vi "Pause.vi"(8 "error in (no error)":errorcluster, 11 "Ismatech 3 Channel Settings In":T1={"VISA resource name"="", "Pump Number"=1, "Channel Number"=0, "Simulated?"=TRUE, "Reverse?"=FALSE} {"Channel Number" min=0 max=3; "Pump Number" min=1 max=9}) -> (0 "error out":errorcluster, 1 "Connection Error":bool, 2 "5 Fails":bool, 3 "Ismatech 3 Channel Settings Out":T1={"VISA resource name"="", "Pump Number"=1, "Channel Number"=0, "Simulated?"=TRUE, "Reverse?"=FALSE} {"Channel Number" min=0 max=3; "Pump Number" min=1 max=9})   [LabVIEW 2018, in "Ismatec 4308.lvlib"]
uses:
  Ismatec 4308.lvlib
  Ismatec 4083.ctl
  support/Support Library.lvlib
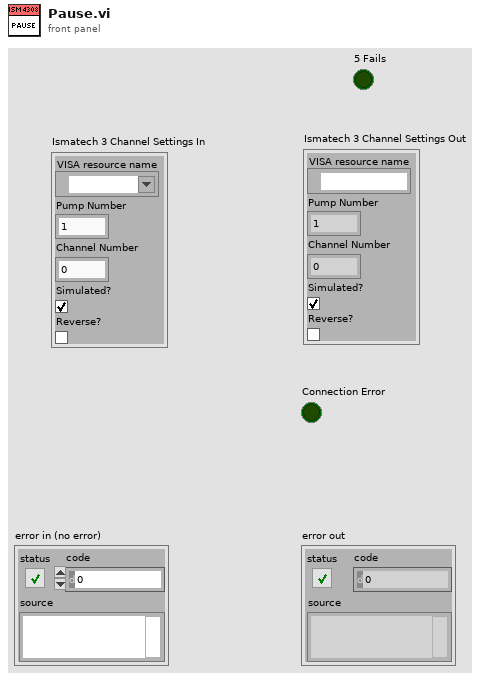
[diagram p1: front panel]
types:
  T1 = typedef "Ismatec 4308.lvlib/Ismatec 4083.ctl" = cluster{"VISA resource name":refnum<visa-resource-name>, "Pump Number":i16, "Channel Number":i16, "Simulated?":bool, "Reverse?":bool}
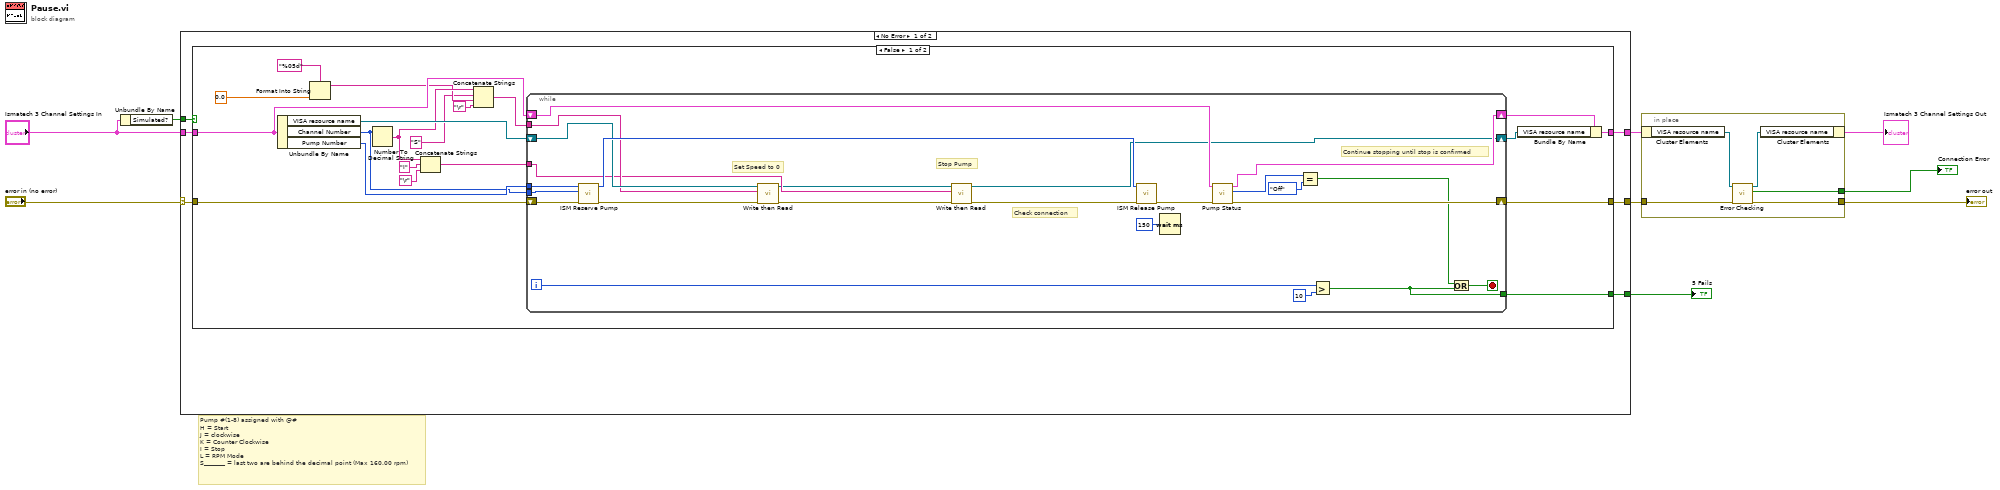
[diagram p0: block diagram]
diagram:
  # "Pump #(1-8) assigned with @#\nH = Start\nJ = clockwise\nK = Counter Clockwise\nI = Stop\nL = RPM Mode\nS_______ = last two are behind the decimal point (Max 160.00 rpm)"
  n1 = Unbundle By Name("Ismatech 3 Channel Settings In") -> ("Simulated?"=w8:bool)
  n2 = case shown="No Error" "error in (no error)" {
    selector: "error in (no error)" -> [w13 w63]
    tunnel: [w12 w62] -> w5
    tunnel: [w11 w63] -> w7
    tunnel: "Ismatech 3 Channel Settings In" -> [w15 w62]
    tunnel: w8 -> [w14 _]
    tunnel: [w10 _] -> w1
    frame No Error {
      n3 = case shown="False" w14 {
        tunnel: w15 -> [w29 w61]
        tunnel: [w35 w61] -> w12
        tunnel: w13 -> [w32 w60]
        tunnel: [w34 w60] -> w11
        tunnel: [w17 _] -> w10
        frame False {
          n4 = Unbundle By Name(w29) -> ("VISA resource name"=w31:refnum<visa-resource-name>, "Channel Number"=w16:i16, "Pump Number"=w18:i16)
          n5 = Format Into String(format string="%05d", 0.0 ("x")) -> (resulting string=w27:string)  [unwired: 2 in, 1 out]
          n6 = Number To Decimal String(number=w16) -> (decimal integer string=w30:string)  [unwired: 1 in]
          n7 = Concatenate Strings(w30, "I", "\r") -> (w19:string)
          n8 = Concatenate Strings(w30, "S" ("string"), w27, "\r") -> (w22:string)
          n9 = while {
            shift-right: [w58] -> w34
            shift-left: w32 -> [w52]
            shift-right: [w38] -> w33
            shift-left: w31 -> [w45]
            shift-right: [w56] -> w28
            shift-left: w29 -> [w57]
            tunnel: w22 -> [w44]
            tunnel: w19 -> [w41]
            tunnel: w18 -> [w53]
            tunnel: [w46] -> w17
            tunnel: w16 -> [w36]
            i -> [w49]
            stop <- w47 stop-if-true
            # "Set Speed to 0"
            # "Check connection"
            # "Stop Pump"
            # "Continue stopping until stop is confirmed"
            n10 = call "ISM Reserve Pump.vi"("error in (no error)"=w52, "ISM Channel # In"=w36, "ISM Pump # In"=w53) -> ("error out"=w43:errorcluster, "ISM Pump # Out"=w51:i32)  [unwired: 7 in]
            n11 = call "Write then Read.vi"("error in"=w43, "write buffer"=w44, "VISA resource name in"=w45) -> ("error out"=w42:errorcluster, "VISA resource name out"=w37:refnum<visa-resource-name>)  [unwired: 6 in, 1 out]
            n12 = call "Write then Read.vi"("error in"=w42, "write buffer"=w41, "VISA resource name in"=w37) -> ("error out"=w39:errorcluster, "VISA resource name out"=w38:refnum<visa-resource-name>)  [unwired: 6 in, 1 out]
            n13 = call "ISM Release Pump.vi"("error in (no error)"=w39, "Pump Number In"=w51) -> ("error out"=w59:errorcluster)  [unwired: 8 in, 1 out]
            n14 = Wait (ms)(milliseconds to wait=u32 150) -> ()  [unwired: 1 out]
            n15 = call "Pump Status.vi"("error in (no error)"=w59, "Ismatech 3 Channel Settings In"=w57) -> ("error out"=w58:errorcluster, "Pump On?"=w55:enum16{"Off", "On", "Not Initialized"}, "Ismatech 3 Channel Settings Out"=w56:T1)  [unwired: 5 in, 2 out]
            n16 = Equal?(x=w55, y=enum16{"Off", "On", "Not Initialized"}."Off") -> (x = y?=w50:bool)
            n17 = Greater?(x=w49, y=10) -> (0:w46:bool)
            n18 = Or(x=w50, y=w46) -> (x .or. y?=w47:bool)
          }
          n19 = Bundle By Name(cluster=w28, "VISA resource name"=w33) -> (w35:T1)
        }
        frame True {
        }
      }
    }
    frame Error {
    }
  }
  "5 Fails" <- w1
  n20 = in-place {
    in-place-border: w7 -> [w68]
    in-place-border: [w67] -> w6
    in-place-border: [w64] -> w4
    n21 = in-place-cluster #1(w5) -> ("VISA resource name"=w66:refnum<visa-resource-name>)
    n22 = call "Error Checking.vi"("error in (no error)"=w68, "VISA resource name"=w66) -> ("error out"=w64:errorcluster, "Connection Error"=w67:bool, "VISA resource name"=w65:refnum<visa-resource-name>)  [unwired: 7 in]
    n23 = in-place-cluster #1("VISA resource name"=w65) -> (→"Ismatech 3 Channel Settings Out":T1)
  }
  "Connection Error" <- w6
  "error out" <- w4
